vi "Get data.vi"() -> ()   [LabVIEW 2018]
uses:
  <vilib>/addons/database/Connection.llb/Conn ObjectReference.ctl
  <vilib>/addons/database/Connection.llb/DB Tools Open Connec (Path).vi
  <vilib>/addons/database/Connection.llb/Conn Execute.vi
  <vilib>/addons/database/Recordset.llb/Rec Fetch Recordset Data (R).vi
  <vilib>/addons/database/Recordset.llb/Rec Destroy - Connection.vi
  <vilib>/addons/database/Recordset.llb/Rec Save Recordset To File (R).vi
  <vilib>/addons/database/_DB Variant To Data/Database Variant To Data.xnode
  <vilib>/addons/database/NI_Database_API.lvlib
panel:
  in  "connection information":path
  in  "table name":string="Test_Results"
  in  "quit":bool
  in  "Export All Data to XML":bool
  in  "File Name":path=path "c:/test data.xml"
  in  "Sort Data":bool
  in  "Sort By":u16(ring) items=["Operator", "Date/Time", "UUT Serial #", "Pass/Fail"]
  in  "Order":u16(ring) items=["Ascending", "Descending"]
  in  "Retrieve Only Failures":bool
  in  "Retrieve All Data":bool
  out "Database Data":i32(listbox)=-1
  out "error out":errorcluster
  out "connection reference out":T1
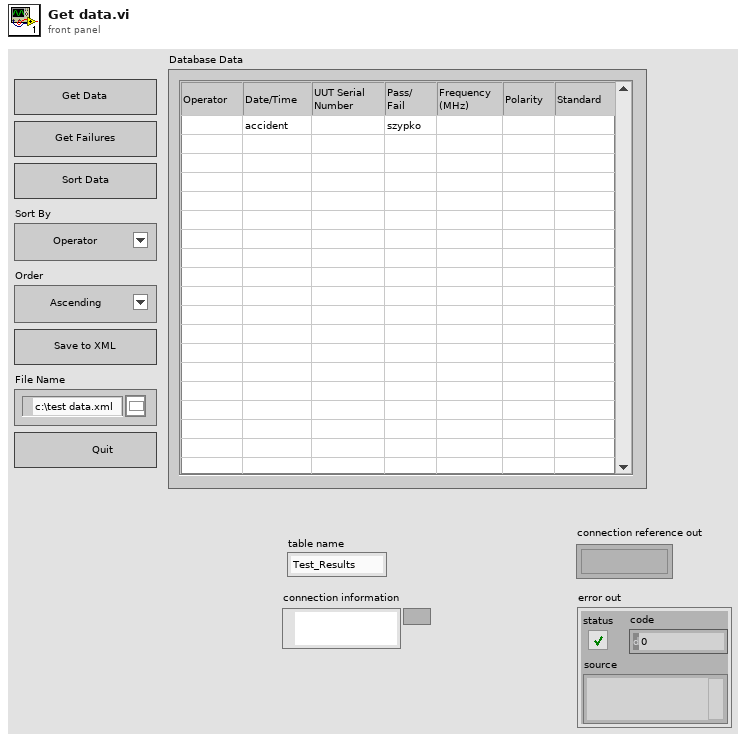
[diagram p1: front panel]
types:
  T1 = typedef "NI_Database_API.lvlib/Conn ObjectReference.ctl" = refnum<k1>
  T2 = typedef "NI_Database_API.lvlib/Rec ObjectReference.ctl" = refnum<k1>
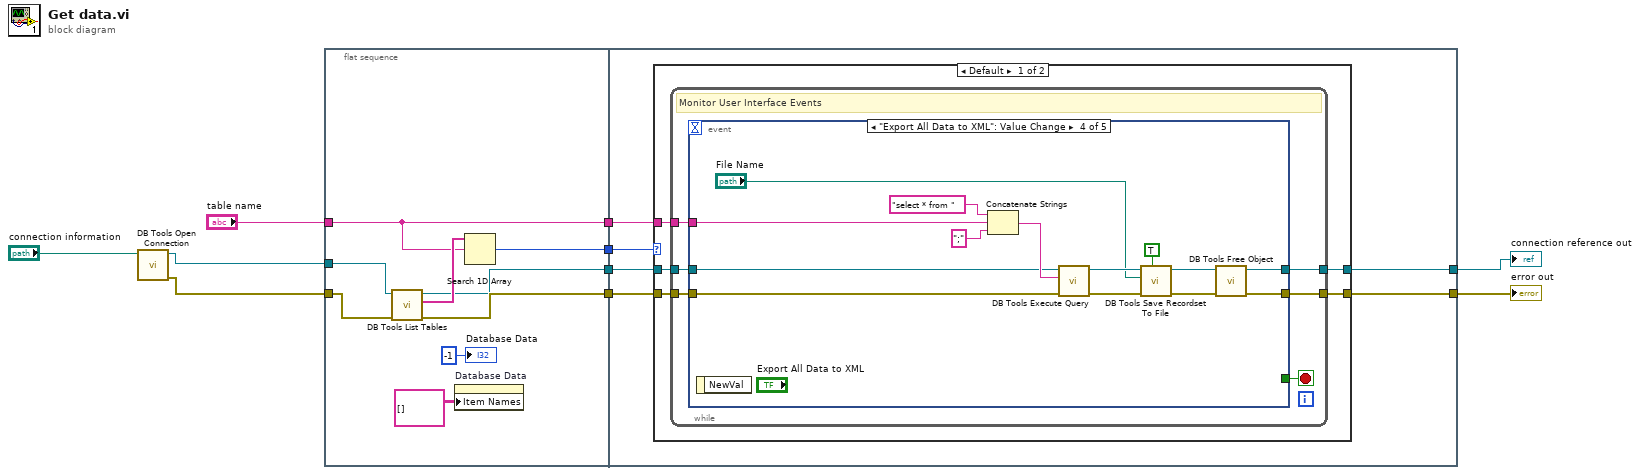
[diagram p0: block diagram]
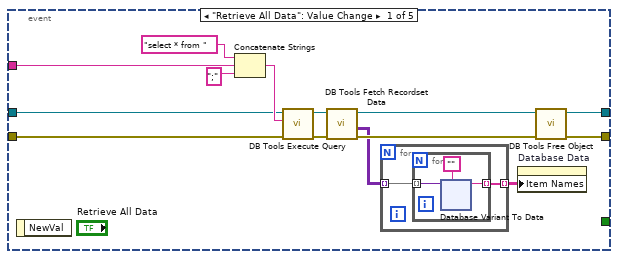
[diagram p2: hidden frame]
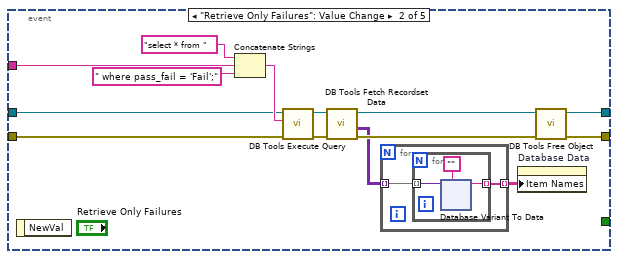
[diagram p3: hidden frame]
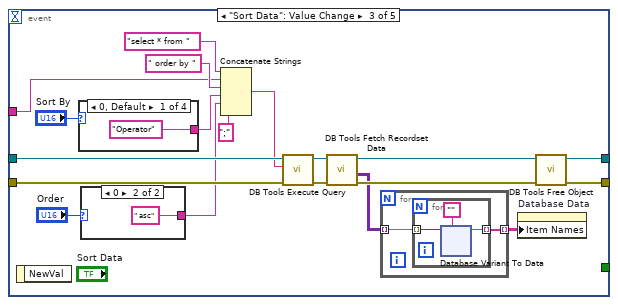
[diagram p4: hidden frame]
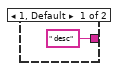
[diagram p5: hidden frame]
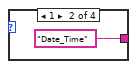
[diagram p6: hidden frame]
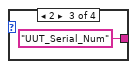
[diagram p7: hidden frame]
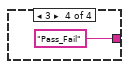
[diagram p8: hidden frame]
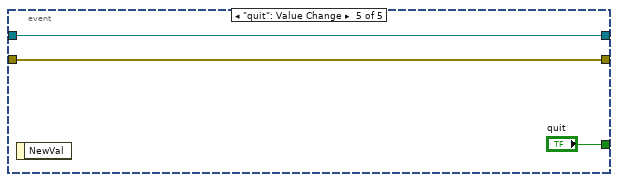
[diagram p9: hidden frame]
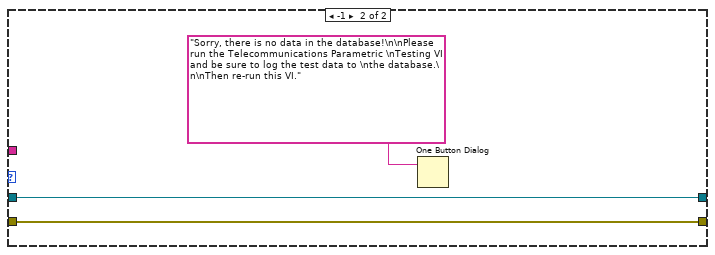
[diagram p10: hidden frame]
diagram:
  n1 = call-poly <vilib>:"DB Tools Open Connection.vi"("connection information"="connection information") -> ("error out"=w1:errorcluster, "connection reference"=w2:T1)  [unwired: 7 in]
  n2 = flat-sequence {
    tunnel: [w16] -> w10
    tunnel: "table name" -> [w12]
    tunnel: w1 -> [w15]
    tunnel: [w14] -> w9
    tunnel: [w13] -> w8
    tunnel: [w12] -> w7
    tunnel: w2 -> [w11]
    tunnel: w10 -> [w25]
    tunnel: w9 -> [w24]
    tunnel: w8 -> [w23]
    tunnel: [w22] -> w4
    tunnel: [w21] -> w5
    tunnel: w7 -> [w20]
    frame #0 {
      n3 = call <vilib>:"DB Tools List Tables.vi"("error in (no error)"=w15, "connection reference"=w11) -> ("error out"=w14:errorcluster, "tables"=w17:string[], "connection reference out"=w13:T1)  [unwired: 3 in]
      n4 = property on="Database Data" class="MCListbox (strict)"("Item Names"=string[][] []) -> ()  [unwired: 2 in, 2 out]
      n5 = Search 1D Array(1D array=w17, element=w12) -> (index of element=w16:i32)  [unwired: 1 in]
      "Database Data" <- -1 ("Database Data")
    }
    frame #1 {
      n6 = case shown="Default" w25 {
        tunnel: w24 -> [w30 w219]
        tunnel: w23 -> [w29 w220]
        tunnel: [w28 w220] -> w22
        tunnel: [w27 w219] -> w21
        tunnel: w20 -> [w26 _]
        frame Default {
          n7 = while {
            tunnel: w30 -> [w35]
            tunnel: w29 -> [w36]
            tunnel: [w33] -> w28
            tunnel: [w32] -> w27
            tunnel: w26 -> [w31]
            stop <- w34 stop-if-true
            # "Monitor User Interface Events"
            n8 = event shown="[3] \"Export All Data to XML\": Value Change" {
              selector: _ -> [_ _ _ _ _]
              dyn-events: _ -> [_ _ _ _ _]
              timeout: _ -> [_ _ _ _ _]
              tunnel: w36 -> [w42 w93 w151 w206 w217]
              tunnel: w35 -> [w41 w92 w150 w205 w216]
              tunnel: [_ _ _ _ "quit"] -> w34
              tunnel: [w39 w90 w148 w203 w217] -> w33
              tunnel: [w40 w91 w149 w204 w216] -> w32
              tunnel: w31 -> [w38 w89 w141 w202 _]
              event "Retrieve All Data": Value Change {
                n9 = event-data() -> ()  [unwired: 1 in, 1 out]
                n10 = Concatenate Strings("select * from " ("SQL query"), w38, ";" ("Substring")) -> (w43:string)
                n11 = call-poly <vilib>:"DB Tools Execute Query.vi"("error in (no error)"=w41, "SQL query"=w43, "connection reference"=w42) -> ("error out"=w46:errorcluster, "recordset reference"=w45:T2)  [unwired: 5 in]
                n12 = call-poly <vilib>:"DB Tools Fetch Recordset Data.vi"("error in (no error)"=w46, "recordset reference"=w45) -> ("error out"=w50:errorcluster, "recordset data"=w47:variant[][], "recordset reference out"=w49:T2)  [unwired: 3 in]
                n13 = for {
                  tunnel: w47 -> [w52] mode=indexing
                  tunnel: [w51] -> w48 mode=indexing
                  n14 = for {
                    tunnel: w52 -> [w55] mode=indexing
                    tunnel: [w54] -> w51 mode=indexing
                    n15 = xnode "Database Variant To Data"("database variant"=w55, "type"="") -> ("data"=w54:string)  [unwired: 1 in, 1 out]
                  }
                }
                n16 = property on="Database Data" class="MCListbox (strict)"("Item Names"=w48) -> ()  [unwired: 2 in, 2 out]
                n17 = call-poly <vilib>:"DB Tools Free Object.vi"("error in (no error)"=w50, "recordset reference"=w49) -> ("error out"=w40:errorcluster, "connection reference"=w39:T1)  [unwired: 8 in]
              }
              event "Retrieve Only Failures": Value Change {
                n18 = event-data() -> ()  [unwired: 1 in, 1 out]
                n19 = Concatenate Strings("select * from " ("SQL query"), w89, " where pass_fail = 'Fail';" ("Substring")) -> (w94:string)
                n20 = call-poly <vilib>:"DB Tools Execute Query.vi"("error in (no error)"=w92, "SQL query"=w94, "connection reference"=w93) -> ("error out"=w97:errorcluster, "recordset reference"=w96:T2)  [unwired: 5 in]
                n21 = call-poly <vilib>:"DB Tools Fetch Recordset Data.vi"("error in (no error)"=w97, "recordset reference"=w96) -> ("error out"=w101:errorcluster, "recordset data"=w98:variant[][], "recordset reference out"=w100:T2)  [unwired: 3 in]
                n22 = for {
                  tunnel: w98 -> [w103] mode=indexing
                  tunnel: [w102] -> w99 mode=indexing
                  n23 = for {
                    tunnel: w103 -> [w106] mode=indexing
                    tunnel: [w105] -> w102 mode=indexing
                    n24 = xnode "Database Variant To Data"("database variant"=w106, "type"="") -> ("data"=w105:string)  [unwired: 1 in, 1 out]
                  }
                }
                n25 = property on="Database Data" class="MCListbox (strict)"("Item Names"=w99) -> ()  [unwired: 2 in, 2 out]
                n26 = call-poly <vilib>:"DB Tools Free Object.vi"("error in (no error)"=w101, "recordset reference"=w100) -> ("error out"=w91:errorcluster, "connection reference"=w90:T1)  [unwired: 8 in]
              }
              event "Sort Data": Value Change {
                n27 = event-data() -> ()  [unwired: 1 in, 1 out]
                n28 = case shown="0, Default" "Sort By" {
                  tunnel: ["Operator" ("Substring") "Date_Time" ("Substring") "UUT_Serial_Num" ("Substring") "Pass_Fail" ("Substring")] -> w144
                  frame 0, Default {
                  }
                  frame 1 {
                  }
                  frame 2 {
                  }
                  frame 3 {
                  }
                }
                n29 = case shown="0" "Order" {
                  tunnel: [" desc" ("Substring") " asc" ("Substring")] -> w139
                  frame 1, Default {
                  }
                  frame 0 {
                  }
                }
                n30 = Concatenate Strings("select * from " ("SQL query"), w141, " order by " ("Substring"), w144, w139, ";" ("Substring")) -> (w142:string)
                n31 = call-poly <vilib>:"DB Tools Execute Query.vi"("error in (no error)"=w150, "SQL query"=w142, "connection reference"=w151) -> ("error out"=w153:errorcluster, "recordset reference"=w152:T2)  [unwired: 5 in]
                n32 = call-poly <vilib>:"DB Tools Fetch Recordset Data.vi"("error in (no error)"=w153, "recordset reference"=w152) -> ("error out"=w157:errorcluster, "recordset data"=w154:variant[][], "recordset reference out"=w156:T2)  [unwired: 3 in]
                n33 = for {
                  tunnel: w154 -> [w165] mode=indexing
                  tunnel: [w164] -> w155 mode=indexing
                  n34 = for {
                    tunnel: w165 -> [w168] mode=indexing
                    tunnel: [w167] -> w164 mode=indexing
                    n35 = xnode "Database Variant To Data"("database variant"=w168, "type"="") -> ("data"=w167:string)  [unwired: 1 in, 1 out]
                  }
                }
                n36 = property on="Database Data" class="MCListbox (strict)"("Item Names"=w155) -> ()  [unwired: 2 in, 2 out]
                n37 = call-poly <vilib>:"DB Tools Free Object.vi"("error in (no error)"=w157, "recordset reference"=w156) -> ("error out"=w149:errorcluster, "connection reference"=w148:T1)  [unwired: 8 in]
              }
              event "Export All Data to XML": Value Change {
                n38 = event-data() -> ()  [unwired: 1 in, 1 out]
                n39 = Concatenate Strings("select * from " ("SQL query"), w202, ";" ("Substring")) -> (w212:string)
                n40 = call-poly <vilib>:"DB Tools Execute Query.vi"("error in (no error)"=w205, "SQL query"=w212, "connection reference"=w206) -> ("error out"=w209:errorcluster, "recordset reference"=w208:T2)  [unwired: 5 in]
                n41 = call-poly <vilib>:"DB Tools Save Recordset To File.vi"("overwrite? (F)"=TRUE ("overwrite? (f)"), "error in (no error)"=w209, "file name"="File Name", "recordset reference"=w208) -> ("error out"=w214:errorcluster, "recordset reference out"=w213:T2)  [unwired: 4 in]
                n42 = call-poly <vilib>:"DB Tools Free Object.vi"("error in (no error)"=w214, "recordset reference"=w213) -> ("error out"=w204:errorcluster, "connection reference"=w203:T1)  [unwired: 8 in]
              }
              event "quit": Value Change {
                n43 = event-data() -> ()  [unwired: 1 in, 1 out]
              }
            }
          }
        }
        frame -1 {
          n44 = One Button Dialog(message="Sorry, there is no data in the database!\n\nPlease run the Telecommunications Parametric \nTesting VI and be sure to log the test data to \nthe database.\n\nThen re-run this VI.") -> ()  [unwired: 1 in, 1 out]
        }
      }
    }
  }
  "connection reference out" <- w4
  "error out" <- w5
